vi "RetaBola.vi"(5 "Meio?":bool=TRUE, 6 "Goal Width":u32, 7 "Field Lenght":u32, 8 "Vy bola":dbl format="%#_13g", 9 "Vx bola":dbl format="%#_13g", 10 "Y bola":dbl format="%#_13g", 11 "X bola":dbl format="%#_13g") -> (0 "Orientação":dbl format="%#_13g", 2 "Y goleiro":dbl format="%#_13g", 3 "X goleiro":dbl format="%#_13g")   [LabVIEW 2017]
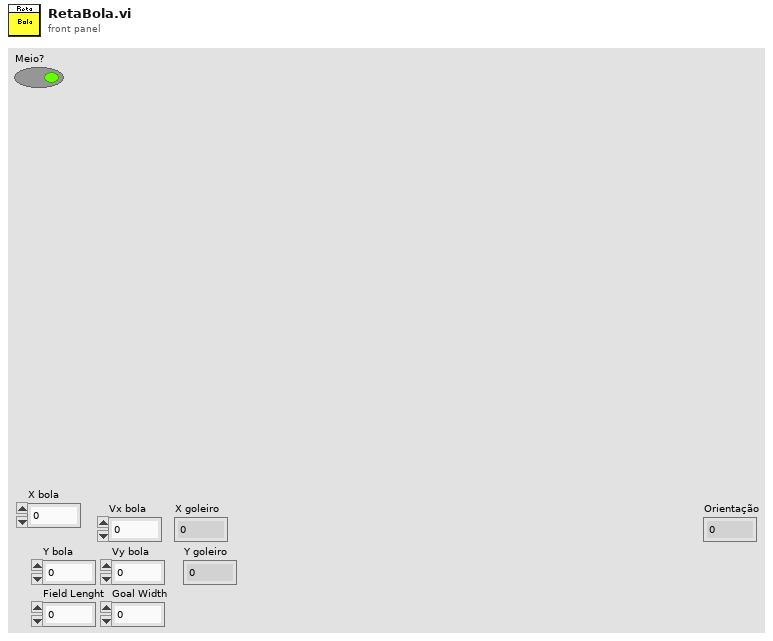
[diagram p1: front panel]
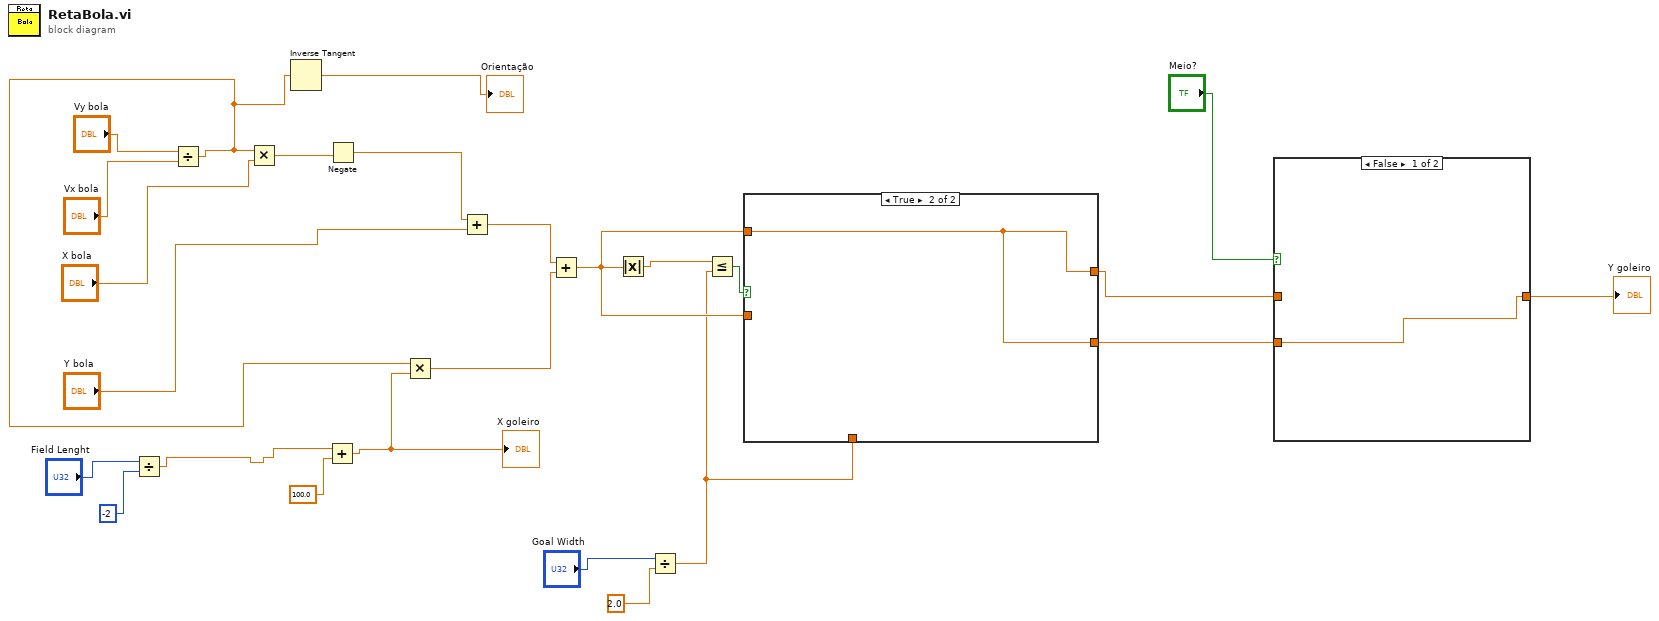
[diagram p0: block diagram]
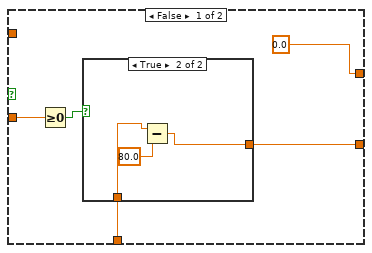
[diagram p3: hidden frame]
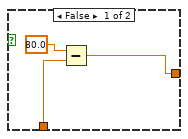
[diagram p4: hidden frame]
diagram:
  n1 = Divide(x="Field Lenght", y=-2 ("Numeric")) -> (x/y=w7:dbl)
  n2 = Divide(x="Vy bola", y="Vx bola") -> (x/y=w9:dbl)
  n3 = Multiply(x=w9, y="X bola") -> (x*y=w21:dbl)
  n4 = Inverse Tangent(1:w9) -> (0:→"Orientação":dbl)
  n5 = Add(x=w7, y=100.0) -> (x+y=w16:dbl)
  "X goleiro" <- w16
  n6 = Negate(x=w21) -> (-x=w20:dbl)
  n7 = Multiply(x=w9, y=w16) -> (x*y=w14:dbl)
  n8 = Add(x=w20, y="Y bola") -> (x+y=w15:dbl)
  n9 = Add(x=w15, y=w14) -> (x+y=w3:dbl)
  n10 = Absolute Value(x=w3) -> (abs(x)=w11:dbl)
  n11 = Divide(x="Goal Width", y=2.0) -> (x/y=w2:dbl)
  n12 = Less Or Equal?(x=w11, y=w2) -> (x <= y?=w10:bool)
  n13 = case shown="True" w10 {
    tunnel: [0.0 w37] -> w5
    tunnel: w3 -> [_ w37]
    tunnel: w3 -> [w29 _]
    tunnel: w2 -> [w27 _]
    tunnel: [w26 w37] -> w1
    frame False {
      n14 = Greater Or Equal To 0?(x=w29) -> (x >= 0?=w28:bool)
      n15 = case shown="True" w28 {
        tunnel: w27 -> [w32 w36]
        tunnel: [w31 w34] -> w26
        frame False {
          n16 = Subtract(x=80.0 ("y"), y=w32) -> (x-y=w31:dbl)
        }
        frame True {
          n17 = Subtract(x=w36, y=80.0 ("x-y")) -> (x-y=w34:dbl)
        }
      }
    }
    frame True {
    }
  }
  n18 = case shown="False" "Meio?" {
    tunnel: w5 -> [_ w39]
    tunnel: [w38 w39] -> w4
    tunnel: w1 -> [w38 _]
    frame False {
    }
    frame True {
    }
  }
  "Y goleiro" <- w4
